vi "Get Cell View .NET.vi"(11 "Cell View in":refnum<class "Cell View.lvclass">) -> (2 "Cell View .NET":refnum<k24>, 3 "Cell View out":refnum<class "Cell View.lvclass">)   [LabVIEW 2024, in "SourceGrid.lvlib" / "Cell View.lvclass"]
uses:
  Cell View.lvclass
  D:/git/Sourcegrid-LabVIEW/dll/SourceGrid.dll
  dll/SourceGrid.dll
  Cell View.lvclass/Cell View.ctl
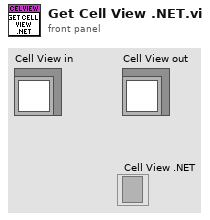
[diagram p1: front panel]
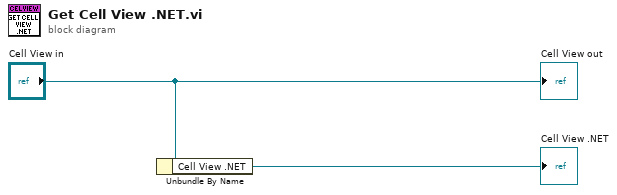
[diagram p0: block diagram]
diagram:
  n1 = Unbundle By Name("Cell View in") -> ("Cell View .NET"=→"Cell View .NET":refnum<k24>)
  "Cell View out" <- "Cell View in"
